vi "CRISTALIZADOR.vi"() -> ()   [LabVIEW 2017]
uses:
  CRISTALIZADOR_datosEnsayo.ctl
  AGILENT 34970/34970_Configuracion.ctl
  CRISTALIZADOR_COMM.ctl
  CRISTALIZADOR_parametrosMedida.ctl
  CRISTALIZADOR_runControl.ctl
  TIMING/Timing_Module Control.ctl
  <vilib>/Utility/error.llb/DialogType.ctl
  IKA_EUROSTAR 60/IKA_Eurostar60.ctl
  AGILENT 34970/34970_CRISTALIZADOR Module.ctl
  FILE/File_Module Control.ctl
  CRISTALIZADOR_GLOBALES.vi
panel:
  out "Temp":string
  out "vNom":string
  out "vReal":string
  out "Par":string
  out "Promedios":i32=1
  out "Ensayo":T1={"Nombre ensayo"="Nombre", "Muestra"="Usuario", "Promedios"=10, "Frecuencia adq(s)"=1.0, "Tiempo medida(min) "=0.0} {"Frecuencia adq(s)" format="%.3f"}
  out "ENABLE":bool
  out "ALARMA":bool
  out "error out":errorcluster
  out "COMMS":T2={"IKA_Eurostar"="", "IKA"=FALSE, "Agilent"="ASRL6::INSTR", "AGL"=FALSE}
  in  "Tab Control":T3(tab)
  out "TEMP":dbl caption="C" format="%.2f"
  in  "Rotador":bool
  in  "Camara":bool
  out "#DATOS":dbl=1.0
  out "FECHA":string
  out "HORA":string
  out "Tiempo total (min)":dbl=10.0
  out "Muestra":string="Muestra"
  out "Ensayo":string="Ensayo"
  out "Muestreo":bool
  out "Error":bool
  out "Tiempo actual (min)":dbl=10.0
  in  "Frecuencia (sec)":dbl=5.0
  in  "Power On Button":bool
  in  "Start Button":bool
  out "Fichero":path
  out "Estado":string
  in  "Abort Button":bool
  out "T1":dbl caption="C" format="%.1f"
  out "T2":dbl caption="C" format="%.1f"
  out "T3":dbl caption="C" format="%.1f"
  out "T4":dbl caption="C" format="%.1f"
  out "Ta":dbl caption="C" format="%.1f"
  out "vSP":dbl caption="rpm" format="%.2f"
  out "VEL":dbl caption="rpm" format="%.2f"
  out "PAR":dbl caption="Ncm" format="%.2f"
  out "tCciclo":dbl caption="s" format="%.3f"
  out "Temperaturas":cluster{dbl[], dbl[]}[](graph)
  out "Rotador":cluster{dbl[], dbl[]}[](graph)
  out "configuration file path":path
  out "Dispositivos":T4=[["Temperatura", "emulsion_entrada", "101", "C", "0.00"], ["Temperatura", "emulsion_salida", "102", "C", "0.00"], ["Temperatura", "agua_entrada", "107", "C", "0.00"], ["Temperatura", "agua_salida", "108", "C", "0.00"], ["Temperatura", "ambiente", "105", "C", "0.00"], ["Presion", "emulsion_entrada", "103", "bar", "0.00"], ["Presion", "emulsion_salida", "109", "bar", "0.00"], ["Presion", "agua_entrada", "110", "bar", "0.00"], ["Presion", "agua_salida", "114", "bar", "0.00"], ["Presion", "", "", "bar", "0.00"], ["Caudal", "caudalimetro", "120", "L/h", "0.00"], ["Caudal", "", "", "L/h", "0.00"], ["Caudal", "", "", "L/h", "0.00"], ["Caudal", "", "", "L/h", "0.00"], ["Caudal", "", "", "L/h", "0.00"]] caption="configuracionCanales"
  out "Datos":T5 {"ROT_TEMPERATURA_C" format="%.2f"; "S5_TEMPERATURA_C" format="%.2f"; "S4_TEMPERATURA_C" format="%.2f"; "S3_TEMPERATURA_C" format="%.2f"; "ROT_PAR_NM" format="%.2f"; "ROT_VELOCIDAD_RPM" format="%.2f"; "ROT_SETPOINT_RPM" format="%.2f"; "S2_TEMPERATURA_C" format="%.2f"; "S1_TEMPERATURA_C" format="%.2f"; "TIEMPO_MIN" format="%.2f"}
  out "numPtos":i32=3600
  out "Array":T5[](array[typedef]) {"ROT_TEMPERATURA_C" format="%.2f"; "S5_TEMPERATURA_C" format="%.2f"; "S4_TEMPERATURA_C" format="%.2f"; "S3_TEMPERATURA_C" format="%.2f"; "ROT_PAR_NM" format="%.2f"; "ROT_VELOCIDAD_RPM" format="%.2f"; "ROT_SETPOINT_RPM" format="%.2f"; "S2_TEMPERATURA_C" format="%.2f"; "S1_TEMPERATURA_C" format="%.2f"; "TIEMPO_MIN" format="%.2f"}
  in  "error in (no error)":errorcluster
  # "TEMPERATURAS"
  # "ROTADOR"
  # "CRISTALIZADOR\n\nFeb.2023 asslcdms v2.0\nLV2017"
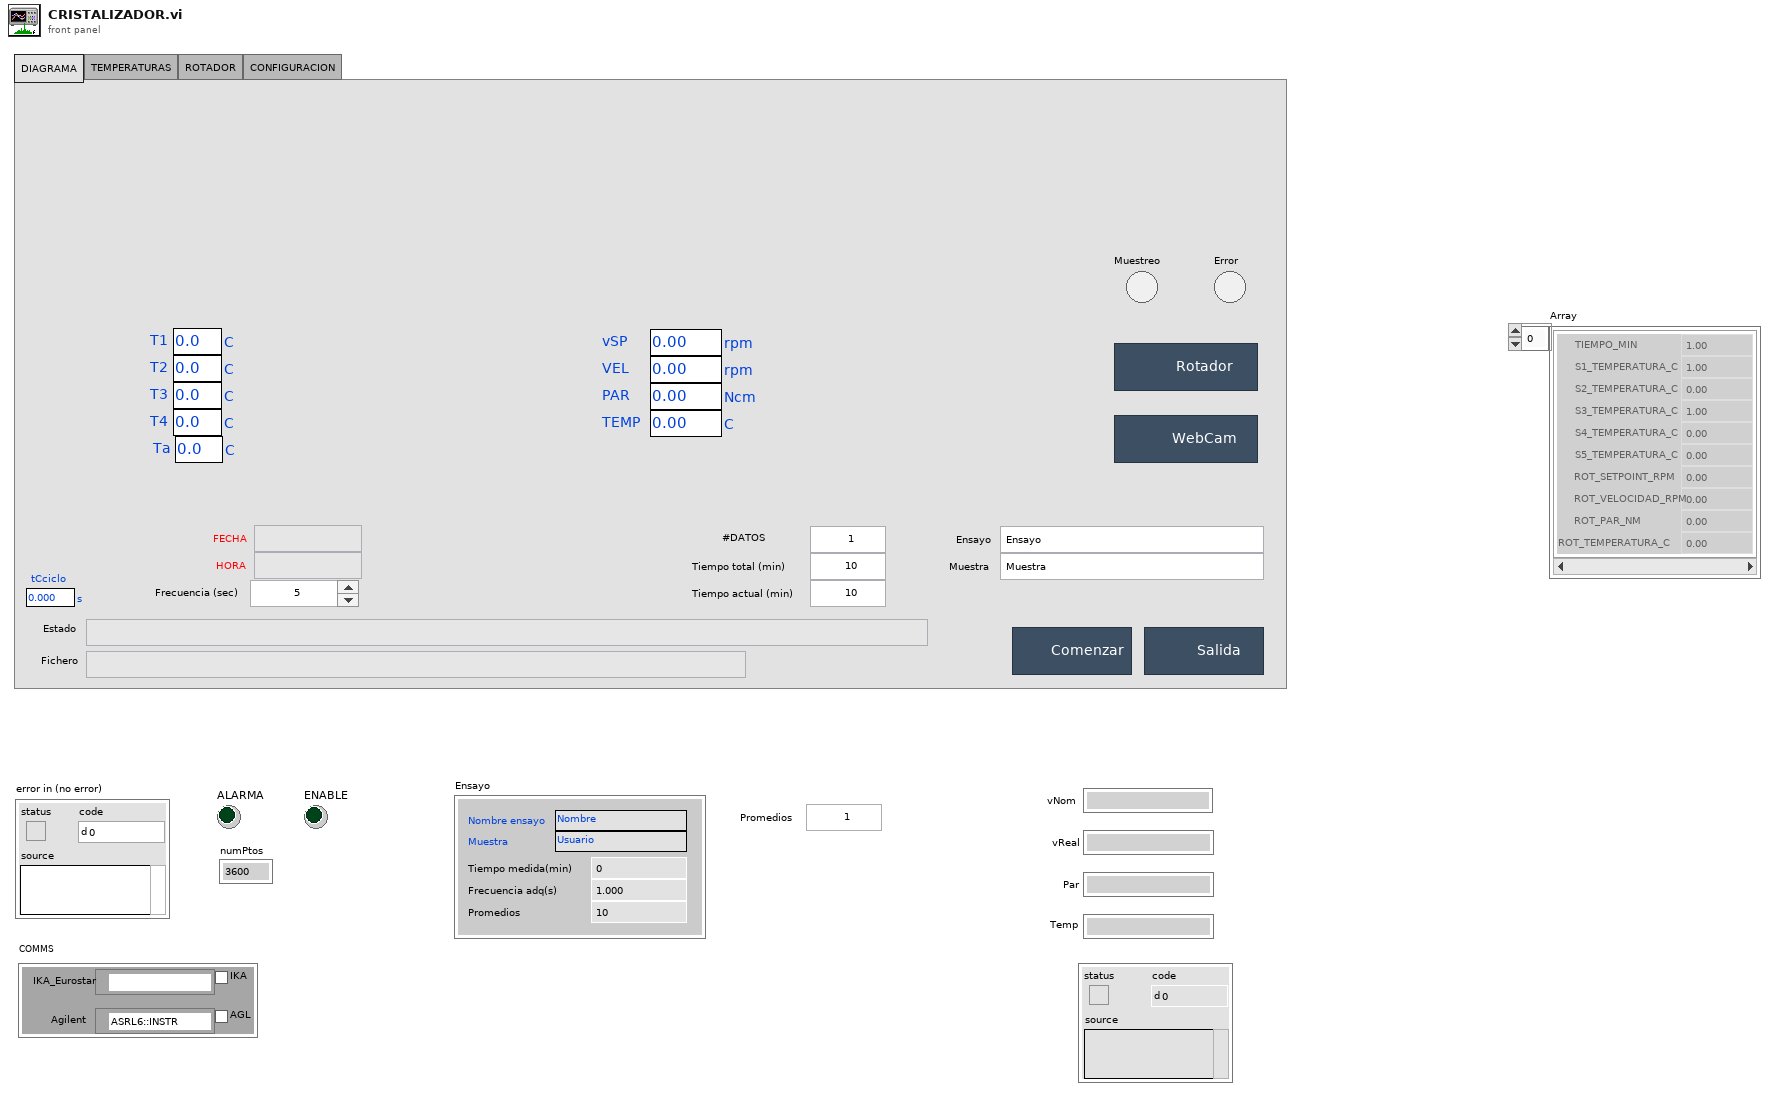
[diagram p1: front panel]
types:
  T1 = typedef "CRISTALIZADOR_parametrosMedida.ctl" = cluster{"Nombre ensayo":string, "Muestra":string, "Promedios":u16, "Frecuencia adq(s)":dbl, "Tiempo medida(min) ":dbl}
  T2 = typedef "CRISTALIZADOR_COMM.ctl" = cluster{"IKA_Eurostar":refnum<visa-resource-name>, "IKA":bool, "Agilent":refnum<visa-resource-name>, "AGL":bool}
  T3 = enum32{"DIAGRAMA", "TEMPERATURAS", "ROTADOR", "CONFIGURACION"}
  T4 = typedef "34970_Configuracion.ctl" = string[][]
  T5 = typedef "CRISTALIZADOR_datosEnsayo.ctl" = cluster{"TIEMPO_MIN":dbl, "S1_TEMPERATURA_C":dbl, "S2_TEMPERATURA_C":dbl, "S3_TEMPERATURA_C":dbl, "S4_TEMPERATURA_C":dbl, "S5_TEMPERATURA_C":dbl, "ROT_SETPOINT_RPM":dbl, "ROT_VELOCIDAD_RPM":dbl, "ROT_PAR_NM":dbl, "ROT_TEMPERATURA_C":dbl}
  T6 = typedef "CRISTALIZADOR_runControl.ctl" = enum16{"INICIALIZAR/CONFIGURAR", "ESPERA COMIENZO", "INICIO DE MEDIDA", "LEER TIEMPO", "LEER AGILENT TEMPERATURAS", "LEER ROTADOR", "GUARDAR DATOS", "ACTUALIZAR GRAFICAS", "SIGUIENTE MUESTRA", "CAMBIOS ROTADOR", "CAMBIOS WEBCAM", "FINALIZAR"}
  T7 = typedef "34970_CRISTALIZADOR Module.ctl" = enum16{"INICIALIZA", "CONFIGURA CANALES", "LECTURA PT100", "LECTURA TERMOPAR", "LECTURA VOLTAJE", "LECTURA CORRIENTE", "SHUTDOWN"}
  T8 = typedef "IKA_Eurostar60.ctl" = enum16{"INICIALIZAR", "READ NOMBRE APARATO", "READ VALOR PT100", "READ VELOCIDAD ACTUAL", "READ PAR DE GIRO ACTUAL", "READ VELOCIDAD NOMINAL", "READ LIMITE PAR DE GIRO", "READ LIMITE VELOCIDAD", "READ VELOCIDAD SEGURIDAD", "SET VELOCIDAD NOMINAL", "SET LIMITE PAR DE GIRO", "SET LIMITE VELOCIDAD", "SET VELOCIDAD SEGURIDAD", "ARRANCAR MOTOR", "DETENER MOTOR", "RESET", "SET SENTIDO DE GIRO", "READ SENTIDO DE GIRO", "FINALIZAR"}
  T9 = typedef "Timing_Module Control.ctl" = enum16{"Initialize Time", "Check Time"}
  T10 = typedef "File_Module Control.ctl" = enum16{"Initialize", "Save Head", "Save Data", "Shutdown"}
  T11 = typedef "DialogType.ctl" = u16
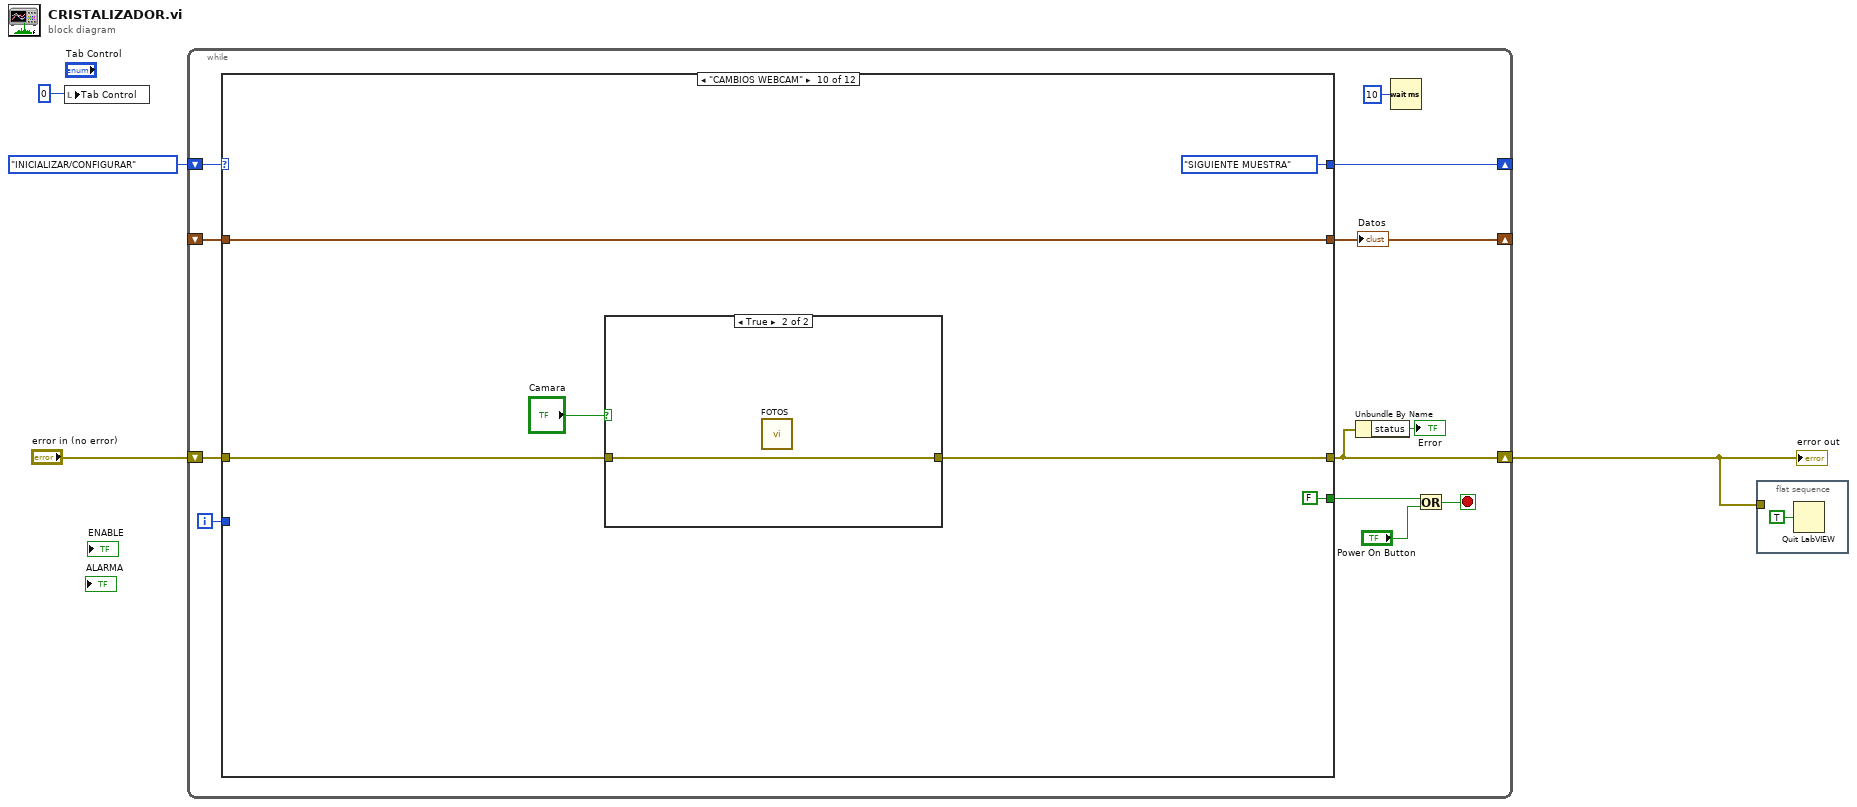
[diagram p0: block diagram]
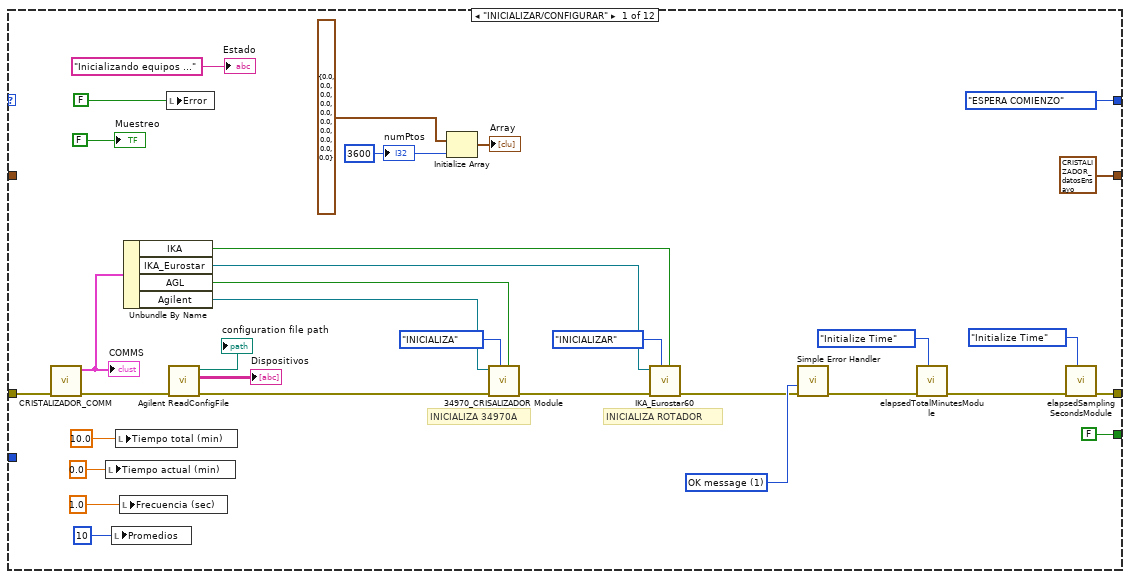
[diagram p2: hidden frame]
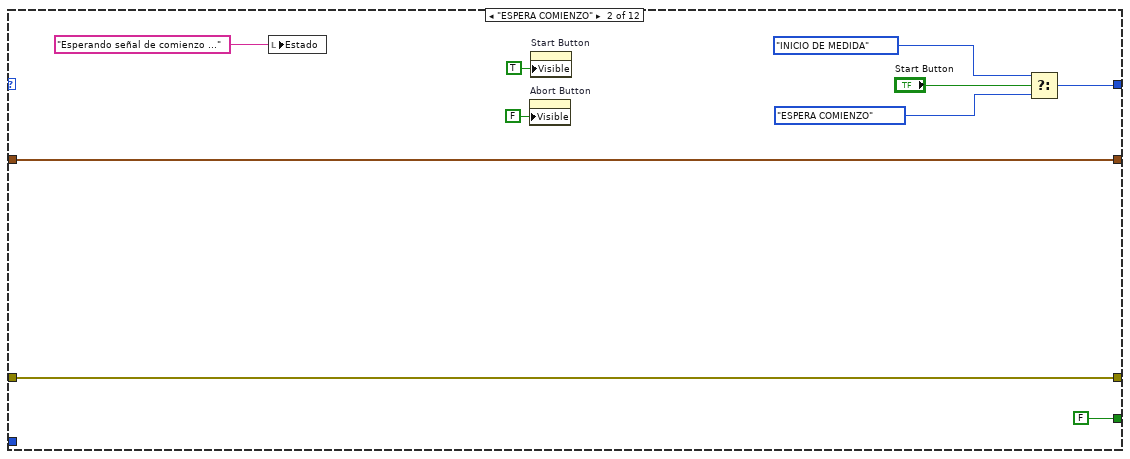
[diagram p3: hidden frame]
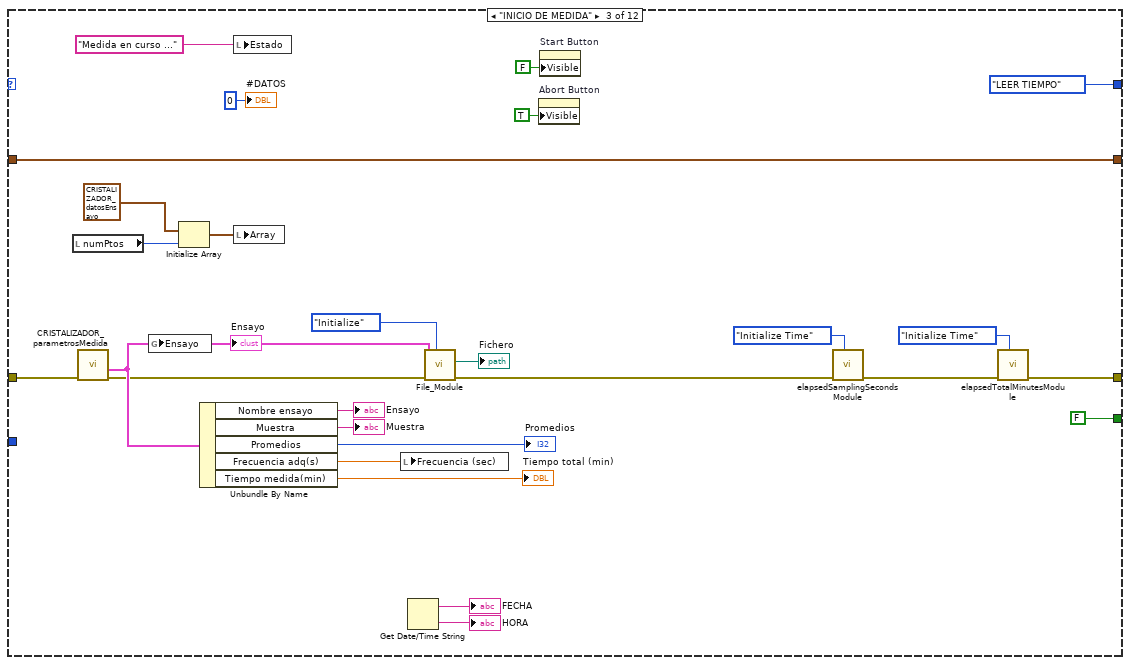
[diagram p4: hidden frame]
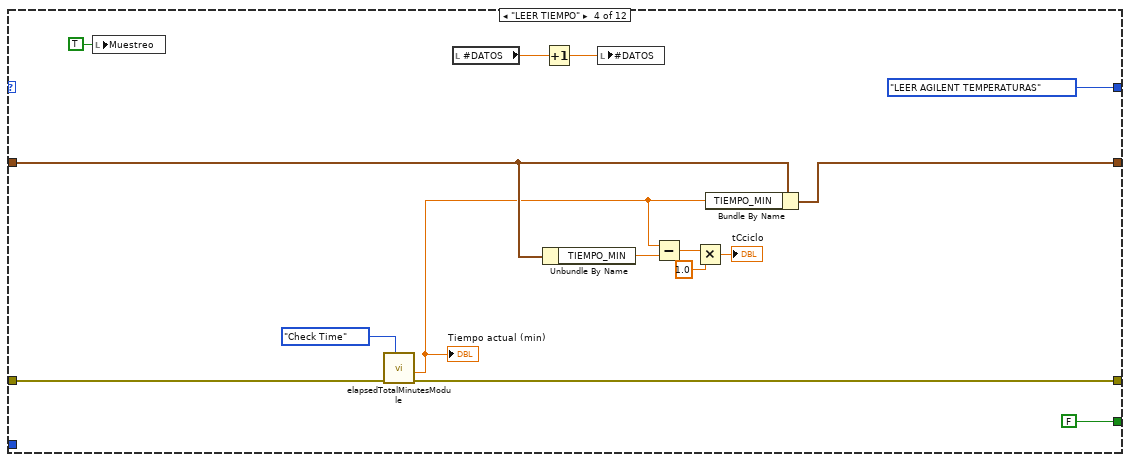
[diagram p5: hidden frame]
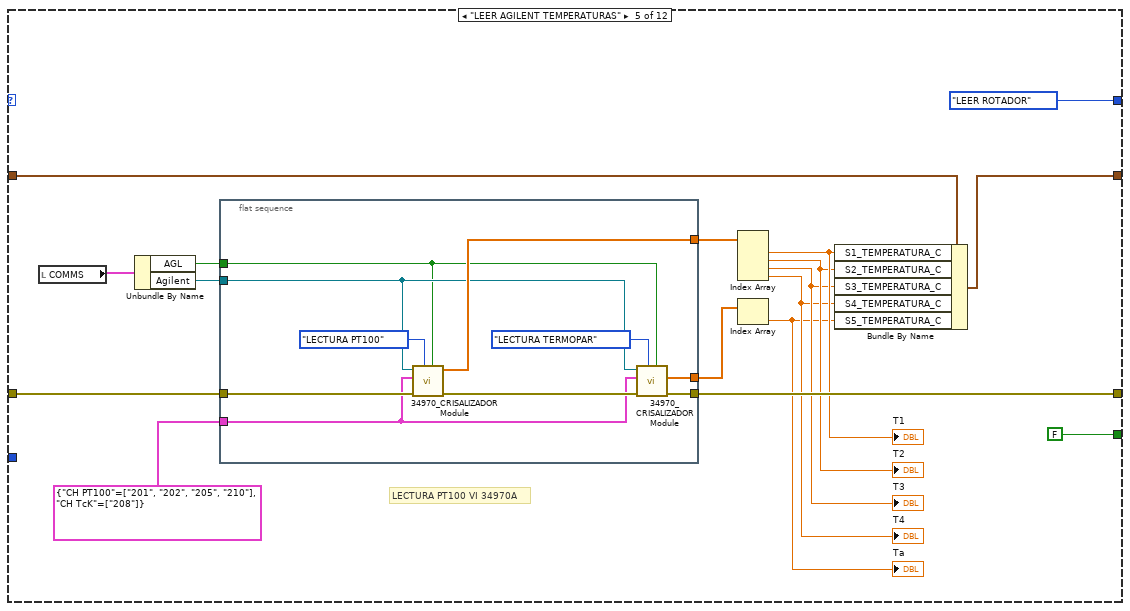
[diagram p6: hidden frame]
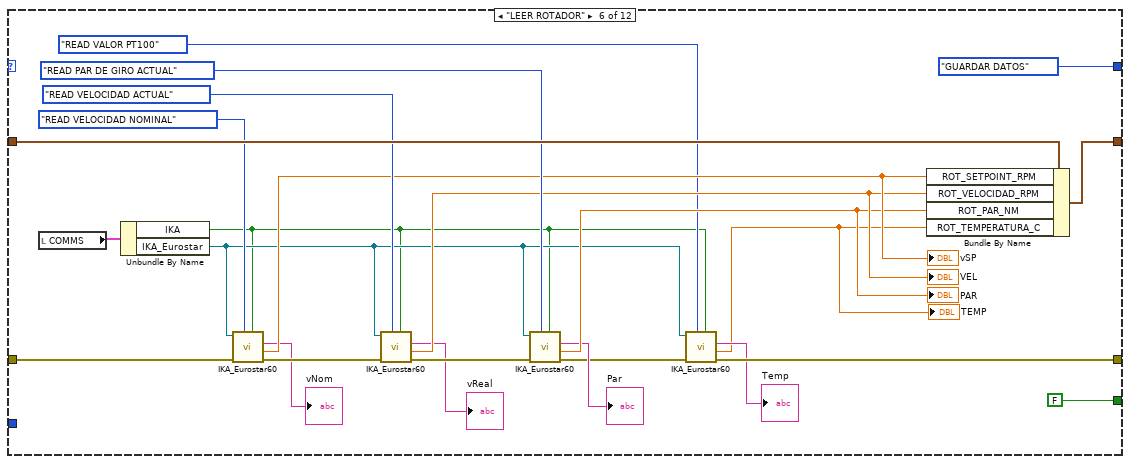
[diagram p7: hidden frame]
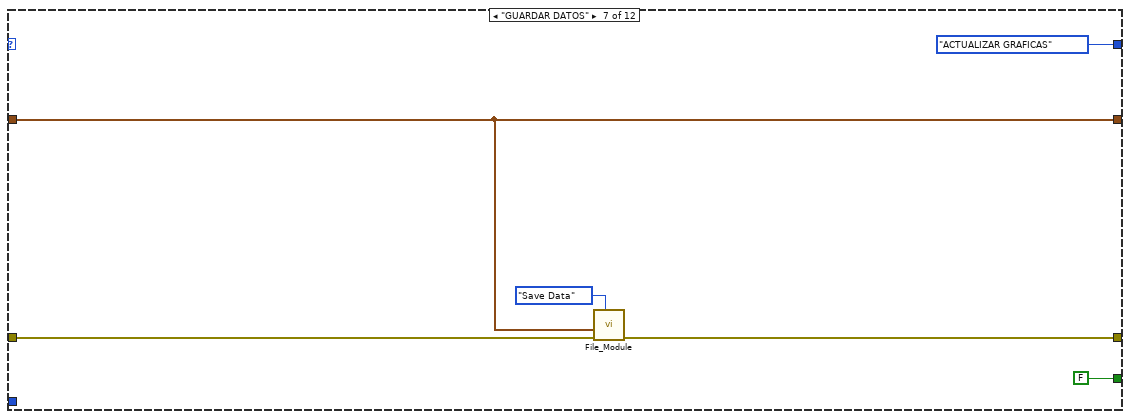
[diagram p8: hidden frame]
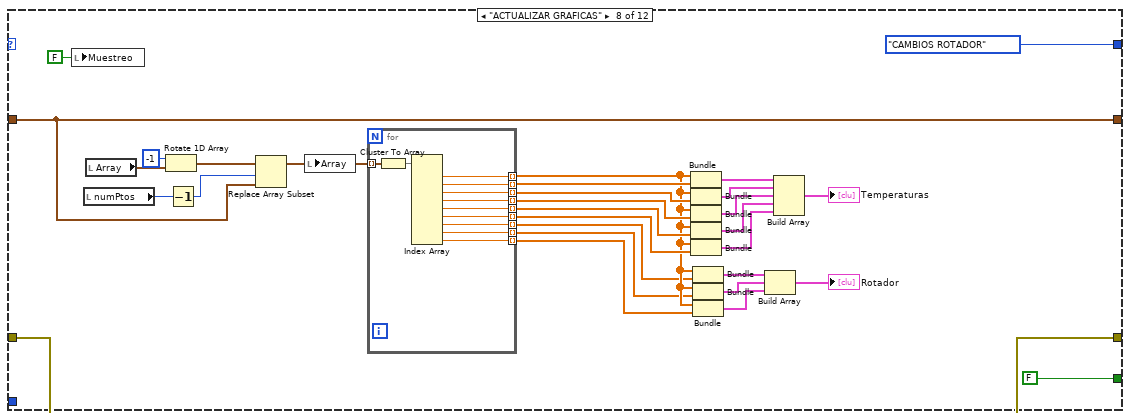
[diagram p9: hidden frame]
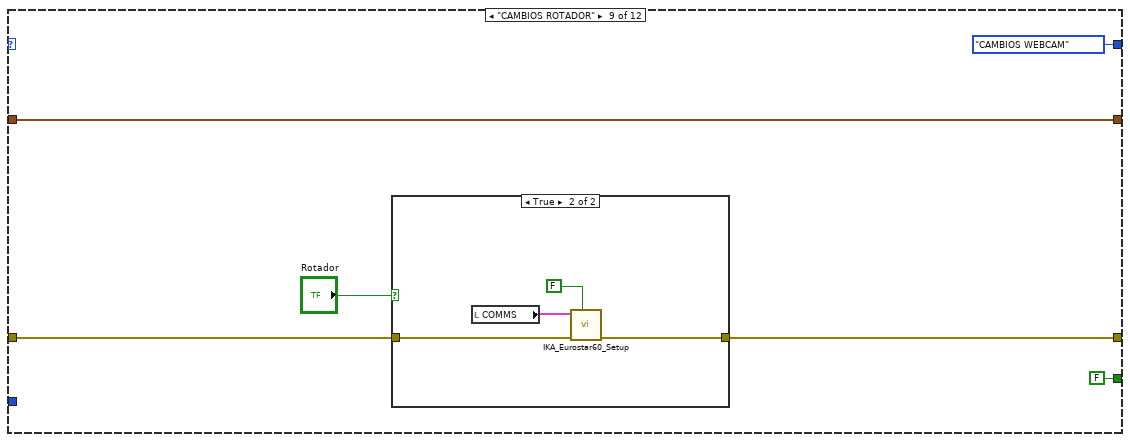
[diagram p10: hidden frame]
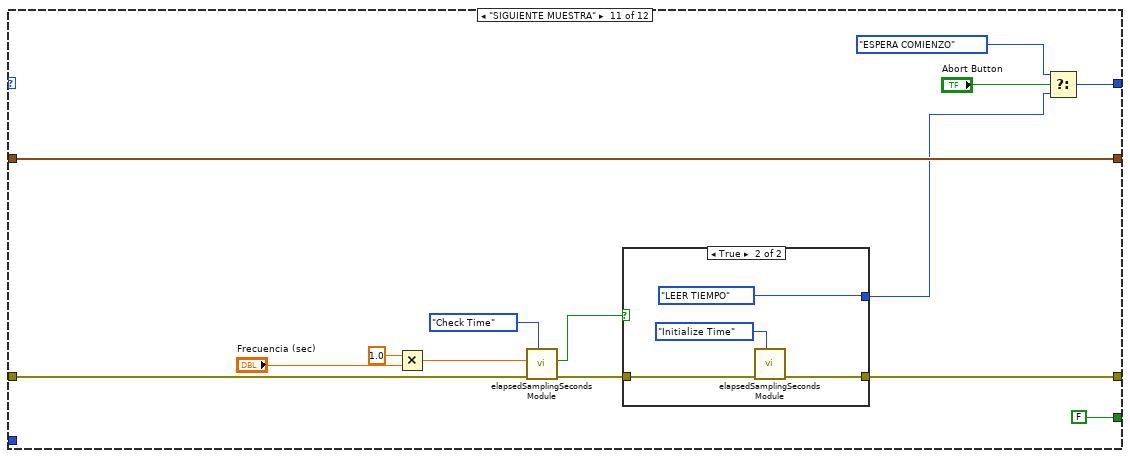
[diagram p13: hidden frame]
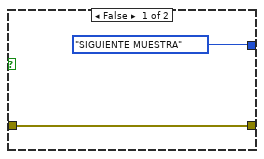
[diagram p14: hidden frame]
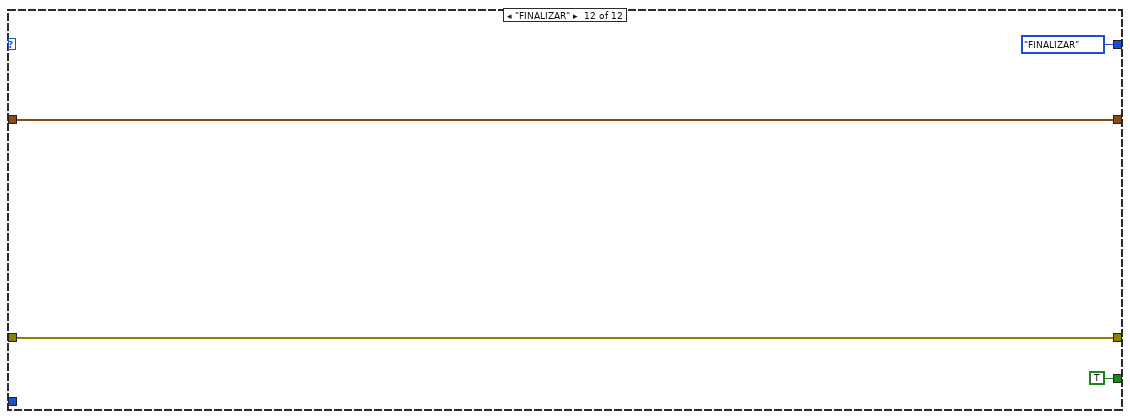
[diagram p15: hidden frame]
diagram:
  n1 = local write "Tab Control"(0 ("n")) -> ()
  n2 = while {
    shift-right: [w8] -> w2
    shift-left: "error in (no error)" -> [w15]
    shift-right: [w13] -> _
    shift-left: CRISTALIZADOR_runControl."INICIALIZAR/CONFIGURAR" ("Beginning State") -> [w14]
    shift-right: [w9] -> _
    shift-left: _ -> [w10]
    i -> [w12]
    stop <- w6 stop-if-true
    n3 = case shown="\"CAMBIOS WEBCAM\"" w14 {
      tunnel: w15 -> [w47 w53 w68 w99 w117 w151 w156 w172 w202 w213 w232 w241]
      tunnel: [w43 w53 w84 w91 w113 w133 w155 w172 w201 w212 w226 w241] -> w8
      tunnel: [FALSE FALSE FALSE FALSE FALSE FALSE FALSE FALSE FALSE FALSE FALSE TRUE] -> w11
      tunnel: [CRISTALIZADOR_runControl."ESPERA COMIENZO" ("Beginning State") w54 CRISTALIZADOR_runControl."LEER TIEMPO" ("Beginning State") CRISTALIZADOR_runControl."LEER AGILENT TEMPERATURAS" ("Beginning State") CRISTALIZADOR_runControl."LEER ROTADOR" ("Beginning State") CRISTALIZADOR_runControl."GUARDAR DATOS" ("Beginning State") CRISTALIZADOR_runControl."ACTUALIZAR GRAFICAS" ("Beginning State") CRISTALIZADOR_runControl."CAMBIOS ROTADOR" ("Beginning State") CRISTALIZADOR_runControl."CAMBIOS WEBCAM" ("Beginning State") CRISTALIZADOR_runControl."SIGUIENTE MUESTRA" ("Beginning State") w219 CRISTALIZADOR_runControl."FINALIZAR" ("Beginning State")] -> w13
      tunnel: w12 -> [_ _ _ _ _ _ _ _ _ _ _ _]
      tunnel: w10 -> [_ w57 w85 w94 w112 w149 w153 w177 w205 w216 w229 w242]
      tunnel: [T5 {"TIEMPO_MIN"=0.0, "S1_TEMPERATURA_C"=0.0, "S2_TEMPERATURA_C"=0.0, "S3_TEMPERATURA_C"=0.0, "S4_TEMPERATURA_C"=0.0, "S5_TEMPERATURA_C"=0.0, "ROT_SETPOINT_RPM"=0.0, "ROT_VELOCIDAD_RPM"=0.0, "ROT_PAR_NM"=0.0, "ROT_TEMPERATURA_C"=0.0} ("Datos") w57 w85 w93 w111 w148 w153 w177 w205 w216 w229 w242] -> w9
      frame "INICIALIZAR/CONFIGURAR" {
        w23 = 3600 ("numPtos")
        w41 = T11 1 items=["no dialog", "OK message", "continue or stop message", "OK message + warnings", "continue/stop + warnings"] ("type of dialog (OK msg:1)")
        # "INICIALIZA ROTADOR"
        # "INICIALIZA 34970A"
        n4 = call "CRISTALIZADOR_COMM.vi"("error in (no error)"=w47) -> ("error out"=w30:errorcluster, "Comunicaciones"=w38:T2)  [unwired: 8 in, 1 out]
        "COMMS" <- w38
        n5 = local write "Tiempo actual (min)"(0.0 ("Tiempo medida")) -> ()
        n6 = local write "Promedios"(u16 10 ("Promedios")) -> ()
        n7 = local write "Tiempo total (min)"(10.0 ("Tiempo medida(min)")) -> ()
        n8 = local write "Frecuencia (sec)"(1.0 ("Tiempo muestreo")) -> ()
        n9 = Unbundle By Name(w38) -> ("IKA"=w18:bool, "IKA_Eurostar"=w17:refnum<visa-resource-name>, "AGL"=w34:bool, "Agilent"=w35:refnum<visa-resource-name>)
        n10 = local write "Error"(FALSE ("Microondas")) -> ()
        n11 = call "Agilent ReadConfigFile.vi"("Error In"=w30) -> ("Error Out"=w29:errorcluster, "Dispositivos"=→"Dispositivos":T4, "configuration file path"=→"configuration file path":path)  [unwired: 7 in]
        n12 = Initialize Array(T5 {"TIEMPO_MIN"=0.0, "S1_TEMPERATURA_C"=0.0, "S2_TEMPERATURA_C"=0.0, "S3_TEMPERATURA_C"=0.0, "S4_TEMPERATURA_C"=0.0, "S5_TEMPERATURA_C"=0.0, "ROT_SETPOINT_RPM"=0.0, "ROT_VELOCIDAD_RPM"=0.0, "ROT_PAR_NM"=0.0, "ROT_TEMPERATURA_C"=0.0} ("Datos"), w23) -> (→"Array":T5[])
        n13 = call "34970_CRISALIZADOR Module.vi"("Agilent 34970A"=w34, "Command"=34970_CRISTALIZADOR_Module."INICIALIZA", "error in (no error)"=w29, "VISA Agilent 34970A"=w35) -> ("error out"=w19:errorcluster)  [unwired: 5 in, 2 out]
        n14 = call "IKA_Eurostar60.vi"("IKAenable"=w18, "Command"=IKA_Eurostar60."INICIALIZAR", "Error in"=w19, "VISA Paar mPDS2000"=w17) -> ("error out"=w20:errorcluster)  [unwired: 5 in, 2 out]
        n15 = call <vilib>:"Simple Error Handler.vi"("type of dialog (OK msg:1)"=w41, "error in (no error)"=w20) -> ("error out"=w42:errorcluster)  [unwired: 3 in, 4 out]
        n16 = call "elapsedTotalMinutesModule.vi"("Command"=Timing_Module_Control."Initialize Time", "error in (no error)"=w42) -> ("error out"=w44:errorcluster)  [unwired: 7 in, 2 out]
        n17 = call "elapsedSamplingSecondsModule.vi"("Command"=Timing_Module_Control."Initialize Time", "error in (no error)"=w44) -> ("error out"=w43:errorcluster)  [unwired: 7 in, 2 out]
        "Estado" <- "Inicializando equipos ..." ("Status")
        "Muestreo" <- FALSE ("Muestreo")
        "numPtos" <- w23
      }
      frame "ESPERA COMIENZO" {
        n18 = local write "Estado"("Esperando señal de comienzo ..." ("Status")) -> ()
        n19 = property on="Abort Button" class="Bool"("Visible"=FALSE) -> ()  [unwired: 2 in, 2 out]
        n20 = property on="Start Button" class="Bool"("Visible"=TRUE) -> ()  [unwired: 2 in, 2 out]
        n21 = Select(t=CRISTALIZADOR_runControl."INICIO DE MEDIDA" ("Beginning State"), s="Start Button", f=CRISTALIZADOR_runControl."ESPERA COMIENZO" ("Beginning State")) -> (s? t:f=w54:T6)
      }
      frame "INICIO DE MEDIDA" {
        n22 = local read "numPtos"() -> (w74:i32)
        n23 = call "CRISTALIZADOR_parametrosMedida.vi"("error in (no error)"=w68) -> ("error out"=w67:errorcluster, "Window"=w69:T1)  [unwired: 8 in, 1 out]
        "Ensayo" <- w69
        n24 = global write "CRISTALIZADOR_GLOBALES.vi" "Ensayo"(w69) -> ()
        n25 = Initialize Array(T5 {"TIEMPO_MIN"=0.0, "S1_TEMPERATURA_C"=0.0, "S2_TEMPERATURA_C"=0.0, "S3_TEMPERATURA_C"=0.0, "S4_TEMPERATURA_C"=0.0, "S5_TEMPERATURA_C"=0.0, "ROT_SETPOINT_RPM"=0.0, "ROT_VELOCIDAD_RPM"=0.0, "ROT_PAR_NM"=0.0, "ROT_TEMPERATURA_C"=0.0} ("Datos"), w74) -> (w73:T5[])
        n26 = Unbundle By Name(w69) -> ("Nombre ensayo"=→"Ensayo":string, "Muestra"=→"Muestra":string, "Promedios"=→"Promedios":u16, "Frecuencia adq(s)"=w61:dbl, "Tiempo medida(min)"=→"Tiempo total (min)":dbl)
        n27 = local write "Estado"("Medida en curso ..." ("Status")) -> ()
        n28 = local write "Array"(w73) -> ()
        n29 = local write "Frecuencia (sec)"(w61) -> ()
        n30 = Get Date/Time String() -> (date string=→"FECHA":string, time string=→"HORA":string)  [unwired: 3 in]
        n31 = call "File_Module.vi"("Command"=File_Module_Control."Initialize", "error in (no error)"=w67, "Window"=w69) -> ("error out"=w78:errorcluster, "selected path"=→"Fichero":path)  [unwired: 7 in]
        n32 = property on="Abort Button" class="Bool"("Visible"=TRUE) -> ()  [unwired: 2 in, 2 out]
        n33 = property on="Start Button" class="Bool"("Visible"=FALSE) -> ()  [unwired: 2 in, 2 out]
        n34 = call "elapsedSamplingSecondsModule.vi"("Command"=Timing_Module_Control."Initialize Time", "error in (no error)"=w78) -> ("error out"=w75:errorcluster)  [unwired: 7 in, 2 out]
        n35 = call "elapsedTotalMinutesModule.vi"("Command"=Timing_Module_Control."Initialize Time", "error in (no error)"=w75) -> ("error out"=w84:errorcluster)  [unwired: 7 in, 2 out]
        "#DATOS" <- 0 ("DATOS")
      }
      frame "LEER TIEMPO" {
        n36 = local write "Muestreo"(TRUE ("Muestreo")) -> ()
        n37 = call "elapsedTotalMinutesModule.vi"("Command"=Timing_Module_Control."Check Time", "error in (no error)"=w99) -> ("error out"=w91:errorcluster, "Elapsed Out"=w90:dbl)  [unwired: 7 in, 1 out]
        "Tiempo actual (min)" <- w90
        n38 = local read "#DATOS"() -> (w87:dbl)
        n39 = Unbundle By Name(w94) -> ("TIEMPO_MIN"=w98:dbl)
        n40 = Increment(x=w87) -> (x+1=w88:dbl)
        n41 = local write "#DATOS"(w88) -> ()
        n42 = Subtract(x=w90, y=w98) -> (x-y=w97:dbl)
        n43 = Multiply(x=w97, y=1.0) -> (x*y=→"tCciclo":dbl)
        n44 = Bundle By Name(cluster=w94, "TIEMPO_MIN"=w90) -> (w93:T5)
      }
      frame "LEER AGILENT TEMPERATURAS" {
        # "LECTURA PT100 VI 34970A"
        n45 = local read "COMMS"() -> (w116:T2)
        n46 = Unbundle By Name(w116) -> ("AGL"=w114:bool, "Agilent"=w115:refnum<visa-resource-name>)
        n47 = flat-sequence {
          tunnel: w117 -> [w127]
          tunnel: w115 -> [w123]
          tunnel: w114 -> [w122]
          tunnel: [w124] -> w113
          tunnel: [w126] -> w110
          tunnel: cluster{"CH PT100":string[], "CH TcK":string[]} {"CH PT100"=["201", "202", "205", "210"], "CH TcK"=["208"]} ("Canales") -> [w121]
          tunnel: [w119] -> w103
          frame #0 {
            n48 = call "34970_CRISALIZADOR Module.vi"("Agilent 34970A"=w122, "Command"=34970_CRISTALIZADOR_Module."LECTURA PT100", "error in (no error)"=w127, "Canales"=w121, "VISA Agilent 34970A"=w123) -> ("error out"=w125:errorcluster, "PT100"=w126:dbl[])  [unwired: 4 in, 1 out]
            n49 = call "34970_CRISALIZADOR Module.vi"("Agilent 34970A"=w122, "Command"=34970_CRISTALIZADOR_Module."LECTURA TERMOPAR", "error in (no error)"=w125, "Canales"=w121, "VISA Agilent 34970A"=w123) -> ("error out"=w124:errorcluster, "TcK"=w119:dbl[])  [unwired: 4 in, 1 out]
          }
        }
        n50 = Index Array(array=w110) -> (element #1=w109:dbl, element #2=w108:dbl, element #3=w107:dbl, element #4=w106:dbl)  [unwired: 4 in]
        "T1" <- w109
        "T2" <- w108
        "T3" <- w107
        "T4" <- w106
        n51 = Index Array(array=w103) -> (element=w102:dbl)  [unwired: 1 in]
        "Ta" <- w102
        n52 = Bundle By Name(cluster=w112, "S1_TEMPERATURA_C"=w109, "S2_TEMPERATURA_C"=w108, "S3_TEMPERATURA_C"=w107, "S4_TEMPERATURA_C"=w106, "S5_TEMPERATURA_C"=w102) -> (w111:T5)
      }
      frame "LEER ROTADOR" {
        n53 = local read "COMMS"() -> (w150:T2)
        n54 = Unbundle By Name(w150) -> ("IKA"=w130:bool, "IKA_Eurostar"=w131:refnum<visa-resource-name>)
        n55 = call "IKA_Eurostar60.vi"("IKAenable"=w130, "Command"=IKA_Eurostar60."READ VELOCIDAD NOMINAL", "Error in"=w151, "VISA Paar mPDS2000"=w131) -> ("error out"=w142:errorcluster, "Read_parametro"=w141:dbl, "read string"=→"vNom":string)  [unwired: 5 in]
        "vSP" <- w141
        n56 = call "IKA_Eurostar60.vi"("IKAenable"=w130, "Command"=IKA_Eurostar60."READ VELOCIDAD ACTUAL", "Error in"=w142, "VISA Paar mPDS2000"=w131) -> ("error out"=w143:errorcluster, "Read_parametro"=w140:dbl, "read string"=→"vReal":string)  [unwired: 5 in]
        "VEL" <- w140
        n57 = call "IKA_Eurostar60.vi"("IKAenable"=w130, "Command"=IKA_Eurostar60."READ PAR DE GIRO ACTUAL", "Error in"=w143, "VISA Paar mPDS2000"=w131) -> ("error out"=w134:errorcluster, "Read_parametro"=w139:dbl, "read string"=→"Par":string)  [unwired: 5 in]
        "PAR" <- w139
        n58 = call "IKA_Eurostar60.vi"("IKAenable"=w130, "Command"=IKA_Eurostar60."READ VALOR PT100", "Error in"=w134, "VISA Paar mPDS2000"=w131) -> ("error out"=w133:errorcluster, "Read_parametro"=w129:dbl, "read string"=→"Temp":string)  [unwired: 5 in]
        "TEMP" <- w129
        n59 = Bundle By Name(cluster=w149, "ROT_SETPOINT_RPM"=w141, "ROT_VELOCIDAD_RPM"=w140, "ROT_PAR_NM"=w139, "ROT_TEMPERATURA_C"=w129) -> (w148:T5)
      }
      frame "GUARDAR DATOS" {
        n60 = call "File_Module.vi"("Command"=File_Module_Control."Save Data", "error in (no error)"=w156, "datosEnsayo"=w153) -> ("error out"=w155:errorcluster)  [unwired: 7 in, 1 out]
      }
      frame "ACTUALIZAR GRAFICAS" {
        n61 = local write "Muestreo"(FALSE ("Muestreo")) -> ()
        n62 = local read "numPtos"() -> (w187:i32)
        n63 = local read "Array"() -> (w180:T5[])
        n64 = Rotate 1D Array(1:w180, 2:-1 ("n")) -> (0:w185:T5[])
        n65 = Decrement(x=w187) -> (x-1=w186:i32)
        n66 = Replace Array Subset(array=w185, new element=w177, index=w186) -> (w179:T5[])
        n67 = local write "Array"(w179) -> ()
        n68 = for {
          tunnel: [w199] -> w181 mode=indexing
          tunnel: [w198] -> w182 mode=indexing
          tunnel: [w197] -> w168 mode=indexing
          tunnel: w179 -> [w195] mode=indexing
          tunnel: [w194] -> w176 mode=indexing
          tunnel: [w193] -> w175 mode=indexing
          tunnel: [w192] -> w171 mode=indexing
          tunnel: [w191] -> w164 mode=indexing
          tunnel: [w190] -> w163 mode=indexing
          tunnel: [w189] -> w162 mode=indexing
          n69 = Cluster To Array(cluster=w195) -> (array=w196:dbl[])
          n70 = Index Array(array=w196) -> (element #1=w197:dbl, element #2=w199:dbl, element #3=w198:dbl, element #4=w194:dbl, element #5=w193:dbl, element #6=w192:dbl, element #7=w191:dbl, element #8=w190:dbl, element #9=w189:dbl)  [unwired: 9 in]
        }
        n71 = Bundle(w168, w181) -> (w183:cluster{dbl[], dbl[]})  [unwired: 1 in]
        n72 = Bundle(w168, w182) -> (w178:cluster{dbl[], dbl[]})  [unwired: 1 in]
        n73 = Bundle(w168, w176) -> (w161:cluster{dbl[], dbl[]})  [unwired: 1 in]
        n74 = Bundle(w168, w175) -> (w160:cluster{dbl[], dbl[]})  [unwired: 1 in]
        n75 = Bundle(w168, w171) -> (w159:cluster{dbl[], dbl[]})  [unwired: 1 in]
        n76 = Bundle(w168, w164) -> (w167:cluster{dbl[], dbl[]})  [unwired: 1 in]
        n77 = Bundle(w168, w163) -> (w166:cluster{dbl[], dbl[]})  [unwired: 1 in]
        n78 = Bundle(w168, w162) -> (w165:cluster{dbl[], dbl[]})  [unwired: 1 in]
        n79 = Build Array(w167, w166, w165) -> (→"Rotador":cluster{dbl[], dbl[]}[])
        n80 = Build Array(w183, w178, w161, w160, w159) -> (→"Temperaturas":cluster{dbl[], dbl[]}[])
      }
      frame "CAMBIOS ROTADOR" {
        n81 = case shown="True" "Rotador" {
          tunnel: w202 -> [w206 w210]
          tunnel: [w206 w209] -> w201
          frame False {
          }
          frame True {
            n82 = local read "COMMS"() -> (w208:T2)
            n83 = call "IKA_Eurostar60_Setup.vi"("Checkbox"=FALSE, "error in"=w210, "COMMS"=w208) -> ("error out"=w209:errorcluster)  [unwired: 8 in]
          }
        }
      }
      frame "CAMBIOS WEBCAM" {
        n84 = case shown="True" "Camara" {
          tunnel: w213 -> [w217 w218]
          tunnel: [w217 w218] -> w212
          frame False {
          }
          frame True {
            n85 = call "FOTOS.vi"() -> ()  [unwired: 12 in]
          }
        }
      }
      frame "SIGUIENTE MUESTRA" {
        n86 = Multiply(x=1.0, y="Frecuencia (sec)") -> (x*y=w224:dbl)
        n87 = call "elapsedSamplingSecondsModule.vi"("Command"=Timing_Module_Control."Check Time", "error in (no error)"=w232, "Time In"=w224) -> ("error out"=w227:errorcluster, "Time Elapsed"=w228:bool)  [unwired: 6 in, 1 out]
        n88 = case shown="True" w228 {
          tunnel: [CRISTALIZADOR_runControl."SIGUIENTE MUESTRA" ("Beginning State") CRISTALIZADOR_runControl."LEER TIEMPO" ("Beginning State")] -> w220
          tunnel: w227 -> [w234 w237]
          tunnel: [w234 w236] -> w226
          frame False {
          }
          frame True {
            n89 = call "elapsedSamplingSecondsModule.vi"("Command"=Timing_Module_Control."Initialize Time", "error in (no error)"=w237) -> ("error out"=w236:errorcluster)  [unwired: 7 in, 2 out]
          }
        }
        n90 = Select(t=CRISTALIZADOR_runControl."ESPERA COMIENZO" ("Beginning State"), s="Abort Button", f=w220) -> (s? t:f=w219:T6)
      }
      frame "FINALIZAR" {
      }
    }
    "Datos" <- w9
    n91 = Unbundle By Name(w8) -> ("status"=→"Error":bool)
    n92 = Wait (ms)(milliseconds to wait=u32 10) -> ()  [unwired: 1 out]
    n93 = Or(x=w11, y="Power On Button") -> (x .or. y?=w6:bool)
  }
  "error out" <- w2
  n94 = flat-sequence {
    tunnel: w2 -> [_]
    frame #0 {
      n95 = Quit LabVIEW(quit? (T)=TRUE) -> ()
    }
  }
